vi "Dialog Tester - Formatting.vi"() -> ()   [LabVIEW 2021]
doc: "<b>TEST VI</b> meant to check the pop ups to verify proper message formatting"
uses:
  Popup/message info--typedef.ctl
  Graphics.ctl
  Custom/Custom - Input (DBL)/Custom - Input (DBL).lvclass
  Custom/Custom - Input (I32)/Custom - Input (I32).lvclass
  Custom/Custom - Input (String)/Custom - Input (String).lvclass
  Custom/Custom - One Button/Custom - One Button.lvclass
  Custom/Custom - Timeout/Custom - Timeout.lvclass
  Custom/Custom - Timeout One Button/Custom - Timeout One Button.lvclass
  Custom/Custom - Timeout Two Button/Custom - Timeout Two Button.lvclass
  Custom/Custom - Two Button/Custom - Two Button.lvclass
  Standard/Input (DBL)/Input (DBL).lvclass
  Pop-Up.lvlib
  Standard/Input (I32)/Input (I32).lvclass
  Standard/Input (String)/Input (String).lvclass
  Standard/One Button/One Button.lvclass
  Standard/Timeout/Timeout.lvclass
  Standard/Timeout One Button/Timeout One Button.lvclass
  Standard/Timeout Two Button/Timeout Two Button.lvclass
  Standard/Two Button/Two Button.lvclass
  Popup/Popup.lvclass
  Theme/Theme.lvclass
panel:
  in  "dark?":bool
  out "iteration":i32
  in  "Pop Up Type":enum16{"Custom", "Standard"}(ring)=enum."Standard"
  in  "Error In":errorcluster
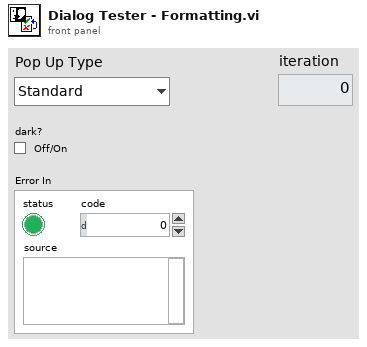
[diagram p1: front panel]
types:
  T1 = typedef "Pop-Up.lvlib/Popup.lvclass/message info--typedef.ctl" = cluster{"Message Height":i32, "Message Width":i32, "Message Location":enum16{"Top", "Bottom", "Right", "Left"}}
  T2 = typedef "Pop-Up.lvlib/Graphics.ctl" = string
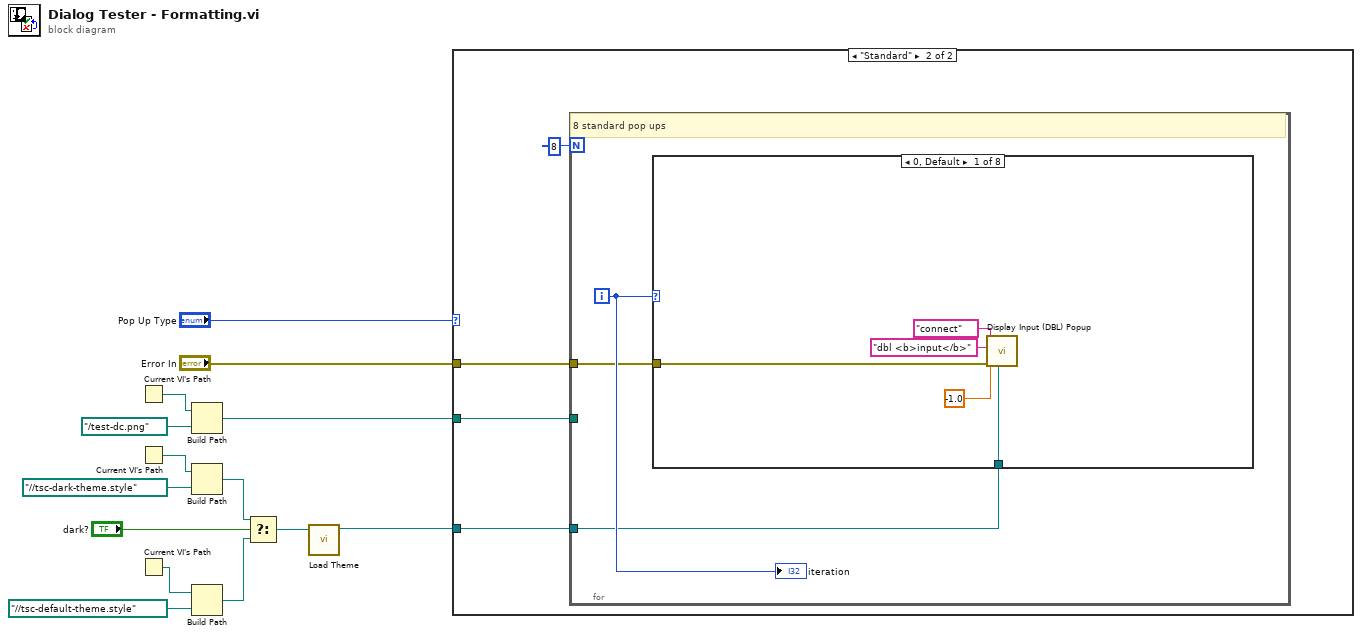
[diagram p0: block diagram]
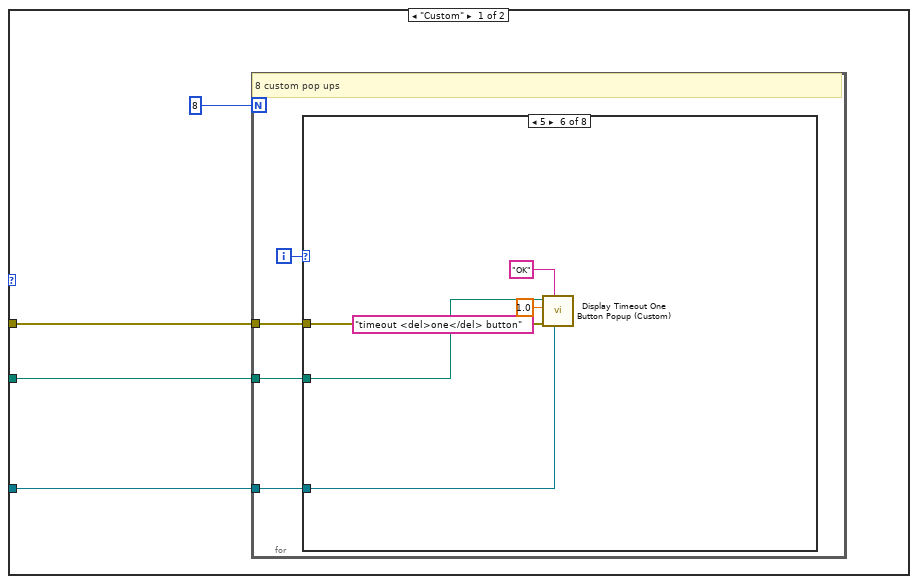
[diagram p2: hidden frame]
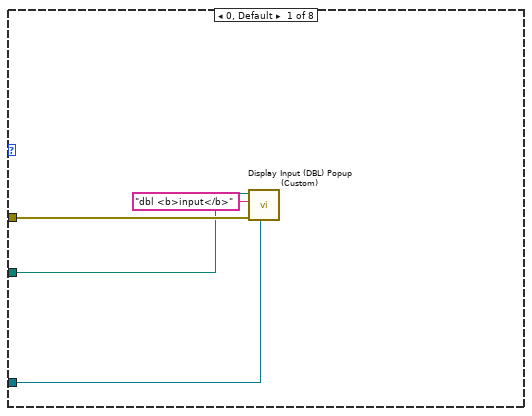
[diagram p3: hidden frame]
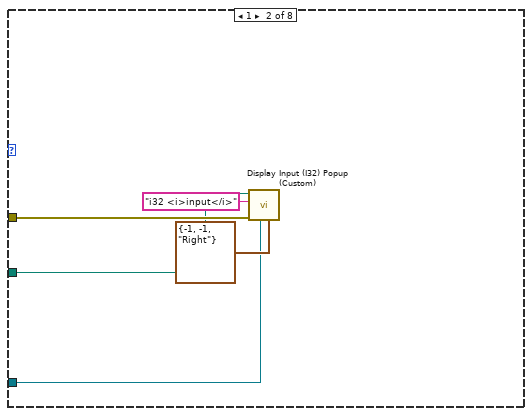
[diagram p4: hidden frame]
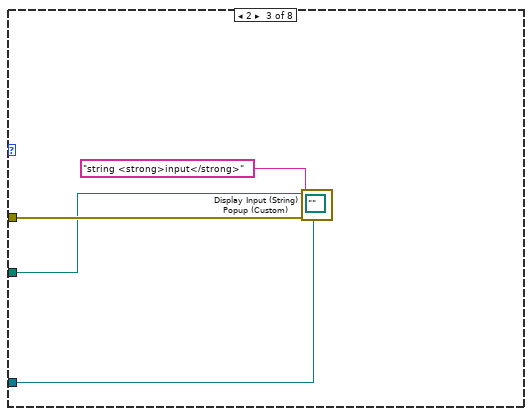
[diagram p5: hidden frame]
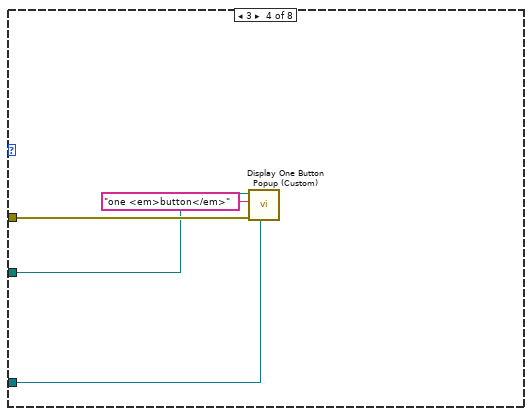
[diagram p6: hidden frame]
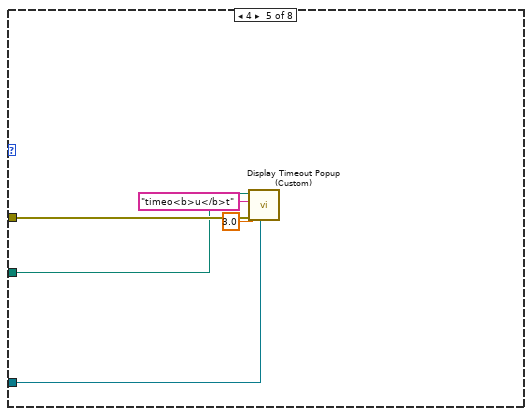
[diagram p7: hidden frame]
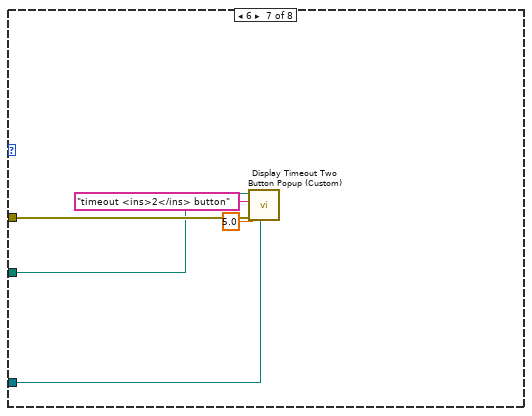
[diagram p8: hidden frame]
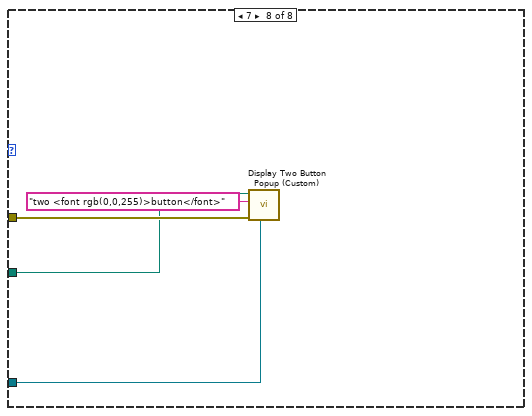
[diagram p9: hidden frame]
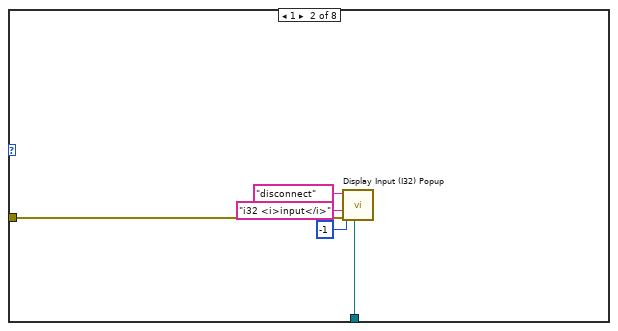
[diagram p10: hidden frame]
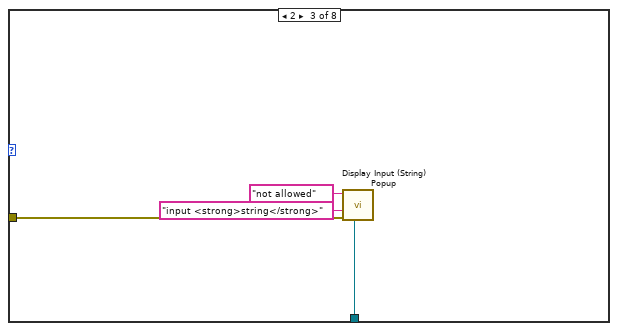
[diagram p11: hidden frame]
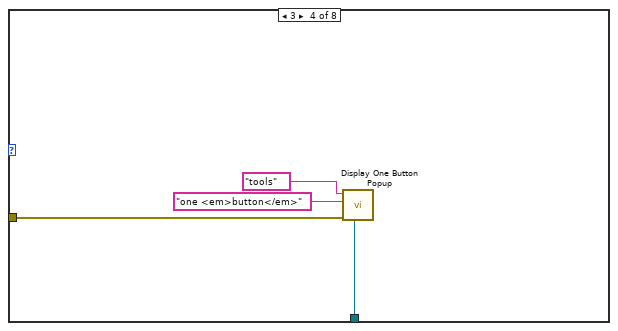
[diagram p12: hidden frame]
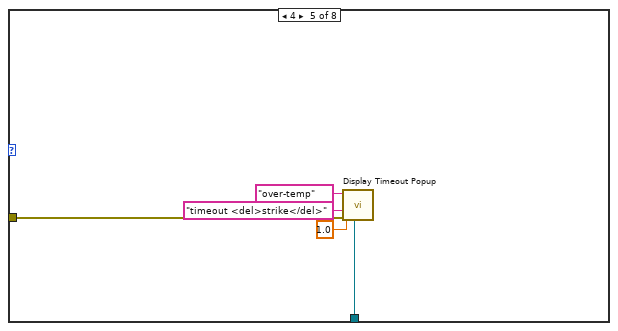
[diagram p13: hidden frame]
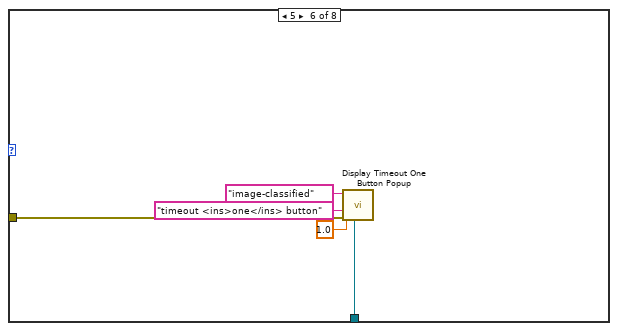
[diagram p14: hidden frame]
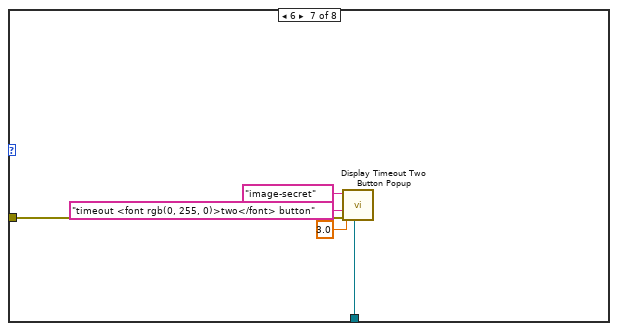
[diagram p15: hidden frame]
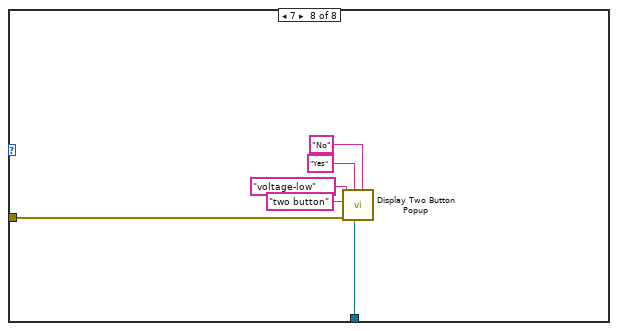
[diagram p16: hidden frame]
diagram:
  n1 = Current VI's Path() -> (path=w14:path)
  n2 = Current VI's Path() -> (path=w8:path)
  n3 = Current VI's Path() -> (path=w2:path)
  n4 = Build Path(base path=w14, name or relative path=path "../test-dc.png") -> (appended path=w12:path)
  n5 = Build Path(base path=w8, name or relative path=path "../../tsc-dark-theme.style") -> (appended path=w7:path)
  n6 = Build Path(base path=w2, name or relative path=path "../../tsc-default-theme.style") -> (appended path=w3:path)
  n7 = Select(t=w7, s="dark?", f=w3) -> (s? t:f=w6:path)
  n8 = call "Load Theme.vi"("File Path"=w6) -> ("Theme"=w1:refnum<class "Theme.lvclass">)  [unwired: 9 in, 1 out]
  n9 = case shown="\"Standard\"" "Pop Up Type" {
    tunnel: w12 -> [w17 w62]
    tunnel: "Error In" -> [w16 w61]
    tunnel: w1 -> [w15 w60]
    frame "Custom" {
      n10 = for {
        N: 8 -> [_]
        tunnel: w17 -> [w21]
        tunnel: w16 -> [w20]
        tunnel: w15 -> [w19]
        i -> [w22]
        # "8 custom pop ups"
        n11 = case shown="5" w22 {
          tunnel: w21 -> [w25 w30 w34 w38 w43 w49 w54 w58]
          tunnel: w20 -> [w26 w31 w35 w39 w44 w50 w55 w59]
          tunnel: w19 -> [w23 w27 w32 w36 w40 w45 w51 w56]
          frame 0, Default {
            n12 = call "Display Input (DBL) Popup (Custom).vi"("Theme"=w23, "Error In"=w26, "Message"="dbl <b>input</b>", "Graphic"=w25) -> ()  [unwired: 6 in, 2 out]
          }
          frame 1 {
            n13 = call "Display Input (I32) Popup (Custom).vi"("Message Size"=T1 {"Message Height"=-1, "Message Width"=-1, "Message Location"=enum."Right"}, "Theme"=w27, "Error In"=w31, "Message"="i32 <i>input</i>", "Graphic"=w30) -> ()  [unwired: 5 in, 2 out]
          }
          frame 2 {
            (unwired) path "" ("appended path")
            n14 = call "Display Input (String) Popup (Custom).vi"("Theme"=w32, "Error In"=w35, "Message"="string <strong>input</strong>", "Graphic"=w34) -> ()  [unwired: 6 in, 2 out]
          }
          frame 3 {
            n15 = call "Display One Button Popup (Custom).vi"("Theme"=w36, "Error In"=w39, "Message"="one <em>button</em>", "Graphic"=w38) -> ()  [unwired: 7 in, 1 out]
          }
          frame 4 {
            n16 = call "Display Timeout Popup (Custom).vi"("Theme"=w40, "Error In"=w44, "Timeout (s)"=3.0, "Message"="timeo<b>u</b>t", "Graphic"=w43) -> ()  [unwired: 6 in, 1 out]
          }
          frame 5 {
            n17 = call "Display Timeout One Button Popup (Custom).vi"("Theme"=w45, "Button Text"="OK", "Error In"=w50, "Timeout (s)"=1.0, "Message"="timeout <del>one</del> button", "Graphic"=w49) -> ()  [unwired: 5 in, 1 out]
          }
          frame 6 {
            n18 = call "Display Timeout Two Button Popup (Custom).vi"("Theme"=w51, "Error In"=w55, "Timeout (s)"=5.0, "Message"="timeout <ins>2</ins> button", "Graphic"=w54) -> ()  [unwired: 5 in, 2 out]
          }
          frame 7 {
            n19 = call "Display Two Button Popup (Custom).vi"("Theme"=w56, "Error In"=w59, "Message"="two <font rgb(0,0,255)>button</font>", "Graphic"=w58) -> ()  [unwired: 6 in, 2 out]
          }
        }
      }
    }
    frame "Standard" {
      n20 = for {
        N: 8 -> [_]
        tunnel: w62 -> [_]
        tunnel: w61 -> [w65]
        tunnel: w60 -> [w64]
        i -> [w66]
        # "8 standard pop ups"
        n21 = case shown="0, Default" w66 {
          tunnel: w65 -> [w71 w76 w80 w84 w89 w94 w99 w105]
          tunnel: w64 -> [w67 w72 w77 w81 w85 w90 w95 w100]
          frame 0, Default {
            n22 = call "Display Input (DBL) Popup.vi"("Theme"=w67, "error in"=w71, "Default Input"=-1.0, "Message"="dbl <b>input</b>", "Graphic"=T2 "connect") -> ()  [unwired: 5 in, 2 out]
          }
          frame 1 {
            n23 = call "Display Input (I32) Popup.vi"("Theme"=w72, "error in"=w76, "Default Input"=-1, "Message"="i32 <i>input</i>", "Graphic"=T2 "disconnect") -> ()  [unwired: 5 in, 2 out]
          }
          frame 2 {
            n24 = call "Display Input (String) Popup.vi"("Theme"=w77, "error in"=w80, "Message"="input <strong>string</strong>", "Graphic"=T2 "not allowed") -> ()  [unwired: 6 in, 2 out]
          }
          frame 3 {
            n25 = call "Display One Button Popup.vi"("Theme"=w81, "error in"=w84, "Message"="one <em>button</em>", "Graphic"=T2 "tools") -> ()  [unwired: 7 in, 1 out]
          }
          frame 4 {
            n26 = call "Display Timeout Popup.vi"("Theme"=w85, "error in"=w89, "Timeout (s)"=1.0, "Message"="timeout <del>strike</del>", "Graphic"=T2 "over-temp") -> ()  [unwired: 6 in, 1 out]
          }
          frame 5 {
            n27 = call "Display Timeout One Button Popup.vi"("Theme"=w90, "error in"=w94, "Timeout (s)"=1.0, "Message"="timeout <ins>one</ins> button", "Graphic"=T2 "image-classified") -> ()  [unwired: 6 in, 1 out]
          }
          frame 6 {
            n28 = call "Display Timeout Two Button Popup.vi"("Theme"=w95, "error in"=w99, "Timeout (s)"=3.0, "Message"="timeout <font rgb(0, 255, 0)>two</font> button", "Graphic"=T2 "image-secret") -> ()  [unwired: 5 in, 2 out]
          }
          frame 7 {
            n29 = call "Display Two Button Popup.vi"("N-Text"="No", "Theme"=w100, "Y-Text"="Yes", "error in"=w105, "Message"="two button", "Graphic"=T2 "voltage-low") -> ()  [unwired: 4 in, 2 out]
          }
        }
        "iteration" <- w66
      }
    }
  }
